vi "Take_snap.vi"(7 "Take_snap":bool, 9 "Camera Session":T1) -> (3 "Number_of_photos 2":i32)   [LabVIEW 2015]
uses:
  <vilib>/userdefined/High Color/IMAQdx.ctl
  <vilib>/vision/driver/NI_Vision_Acquisition_Software.lvlib
panel:
  in  "Number_of_photos":i32
  in  "Boolean 3":bool
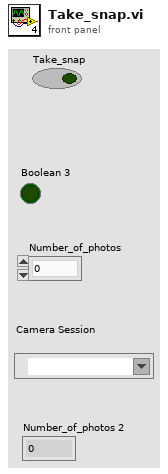
[diagram p1: front panel]
types:
  T1 = typedef "IMAQdx.ctl" = refnum<k21>
  T2 = typedef "IMAQ Image.ctl" = refnum<image>
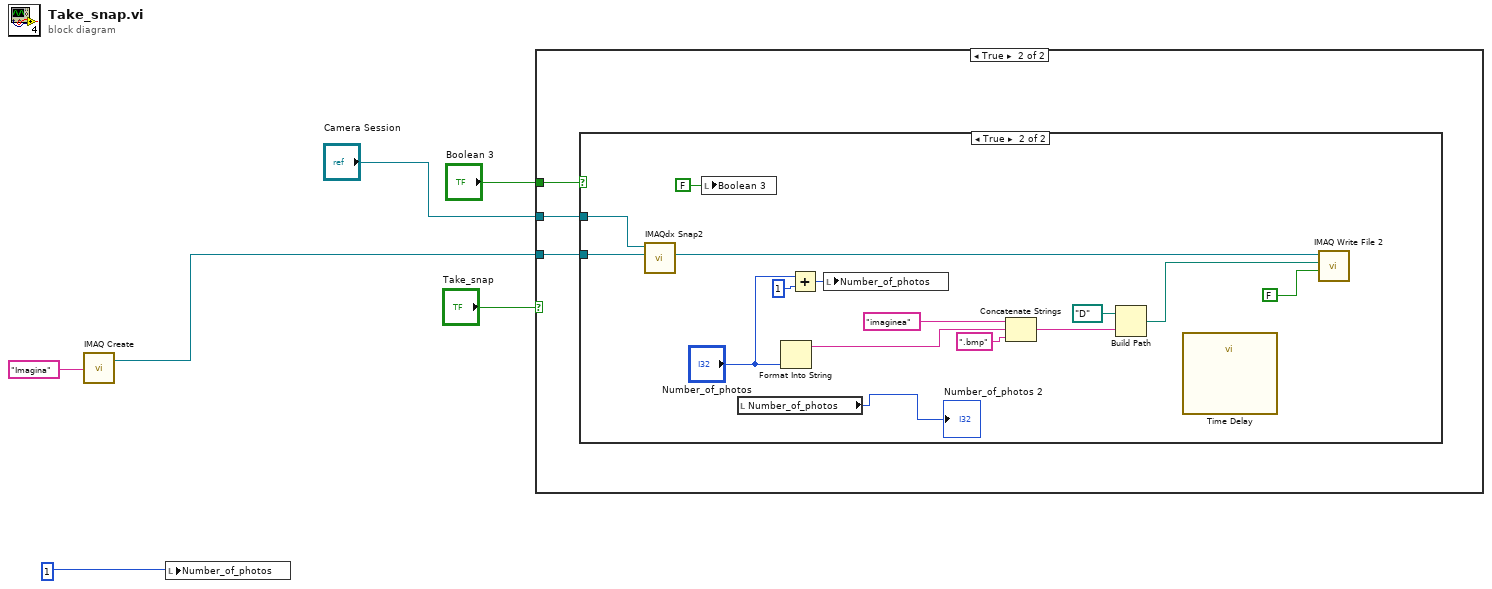
[diagram p0: block diagram]
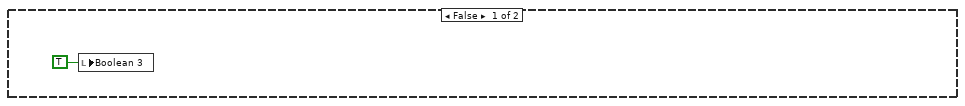
[diagram p2: hidden frame]
diagram:
  n1 = call "IMAQ Create"("Image Name"="Imagina") -> ("New Image"=w5:T2)  [unwired: 4 in, 1 out]
  n2 = local write "Number_of_photos"(1 ("Numeric")) -> ()
  n3 = case shown="True" "Take_snap" {
    tunnel: "Boolean 3" -> [_ w10]
    tunnel: "Camera Session" -> [_ w9]
    tunnel: w5 -> [_ w8]
    frame False {
      n4 = local write "Boolean 3"(TRUE) -> ()
    }
    frame True {
      n5 = case shown="True" w10 {
        tunnel: w9 -> [_ w24]
        tunnel: w8 -> [_ w23]
        frame False {
        }
        frame True {
          n6 = call <vilib>:"IMAQdx Snap2.vi"("Image In"=w23, "Session In"=w24) -> ("Image Out"=w18:T2)  [unwired: 7 in, 2 out]
          n7 = local write "Boolean 3"(FALSE) -> ()
          n8 = local read "Number_of_photos"() -> (→"Number_of_photos 2":i32)
          n9 = Format Into String("Number_of_photos") -> (resulting string=w21:string)  [unwired: 3 in, 1 out]
          n10 = Add(x="Number_of_photos", y=1) -> (x+y=w14:i32)
          n11 = local write "Number_of_photos"(w14) -> ()
          n12 = Concatenate Strings("imaginea" ("string"), w21, ".bmp" ("string")) -> (w19:string)
          n13 = Build Path(base path=path "D:/", name or relative path=w19) -> (appended path=w17:path)
          n14 = call "Time Delay"() -> ()  [unwired: 11 in, 1 out]
          n15 = call-poly "IMAQ Write File 2"("Compress? (N)"=FALSE, "File Path"=w17, "Image"=w18) -> ()  [unwired: 7 in, 2 out]
        }
      }
    }
  }
